vi "GPIB Write Read.vi"(0 "GPIB address":string, 1 "Action":enum16{"Write", "Read", "Write & Read"}(ring), 2 "String to Write":string, 3 "error in (no error)":errorcluster, 4 "wait (mS)":u32) -> (5 "String Read":string, 6 "error out":errorcluster)   [LabVIEW 2019]
doc: "Does a write, read or an uninterrupted write/read since not reentrant.\nAction: 0=Write, 1=Read, 2=Write followed by Read\nScott Hannahs, NHMFL-FSU, December 1995"
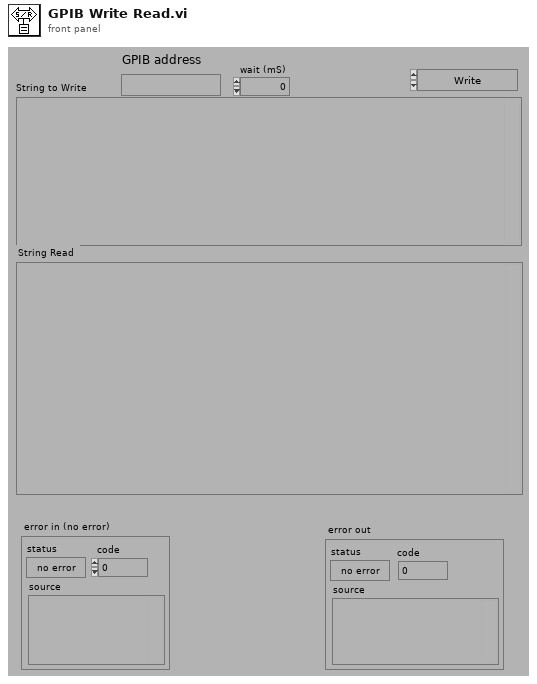
[diagram p1: front panel]
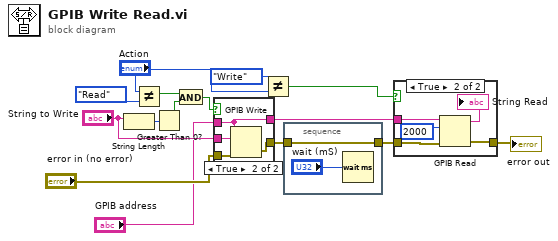
[diagram p0: block diagram]
diagram:
  n1 = String Length(string="String to Write") -> (length=w8:i32)
  n2 = Not Equal?(x="Action", y=enum16{"Write", "Read", "Write & Read"}."Read") -> (x != y?=w11:bool)
  n3 = Greater Than 0?(x=w8) -> (x > 0?=w7:bool)
  n4 = And(x=w11, y=w7) -> (x .and. y?=w9:bool)
  n5 = case shown="True" w9 {
    tunnel: "GPIB address" -> [w17 w19]
    tunnel: [w17 w19] -> w13
    tunnel: [w16 w21] -> w3
    tunnel: "error in (no error)" -> [w16 w20]
    tunnel: "String to Write" -> [_ w18]
    frame False {
    }
    frame True {
      n6 = GPIB Write(0:w19, 1:w18, 3:w20) -> (6:w21:errorcluster)  [unwired: 2 in, 1 out]
    }
  }
  n7 = Not Equal?(x=enum16{"Write", "Read", "Write & Read"}."Write" ("y"), y="Action") -> (x != y?=w10:bool)
  n8 = stacked-sequence {
    tunnel: [w22] -> w2
    tunnel: w3 -> [w22]
    frame #0 {
      n9 = Wait (ms)(milliseconds to wait="wait (mS)") -> ()  [unwired: 1 out]
    }
  }
  n10 = case shown="True" w10 {
    tunnel: [w24 w27] -> w15
    tunnel: w13 -> [_ w29]
    tunnel: w2 -> [w24 w26]
    frame False {
    }
    frame True {
      n11 = GPIB Read(0:w29, 1:2000, 3:w26) -> (5:→"String Read":string, 7:w27:errorcluster)  [unwired: 2 in, 1 out]
    }
  }
  "error out" <- w15
